vi "Get Service Description.vi"(0 "Housekeeping in":refnum<class "Housekeeping.lvclass">, 11 "error in (no error)":errorcluster) -> (4 "Housekeeping out":refnum<class "Housekeeping.lvclass">, 6 "Service Description":string, 15 "error out":errorcluster)   [LabVIEW 2023, in "Room Service Types.lvlib" / "Housekeeping.lvclass"]
uses:
  Housekeeping.lvclass
  Housekeeping.lvclass/Housekeeping.ctl
  Room Service Base/Room Service Base.lvclass
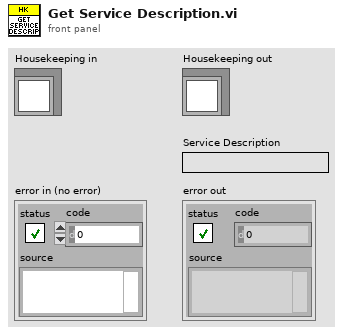
[diagram p1: front panel]
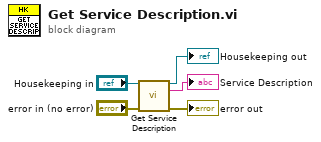
[diagram p0: block diagram]
diagram:
  n1 = call-parent "Get Service Description.vi"("Room Service Base in"="Housekeeping in", "error in (no error)"="error in (no error)") -> ("Room Service Base out"=→"Housekeeping out":refnum<class "Housekeeping.lvclass">, "Service Description"=→"Service Description":string, "error out"=→"error out":errorcluster)  [unwired: 11 in]
